vi "Save Data To File.vi"(7 "Data Type (0: Limit Test Data)":i32(ring) items=["Limit Test Data", "Math Expression Data", "Sense Data", "All Data"], 8 "error in (no error)":errorcluster, 9 "File Name":string, 10 "Channel (1: Channel 1)":i32(ring)=1 items=["Channel 1"=1], 11 "VISA resource name":refnum<visa-resource-name>) -> (0 "error out":errorcluster, 3 "VISA resource name out":refnum<visa-resource-name>)   [LabVIEW 2012, in "Keysight B2980 Series.lvlib"]
doc: "Saves the limit test data, math expression result data, sense data, or all of these data for the specified channel to the specified file in the current directory."
uses:
  Keysight B2980 Series.lvlib
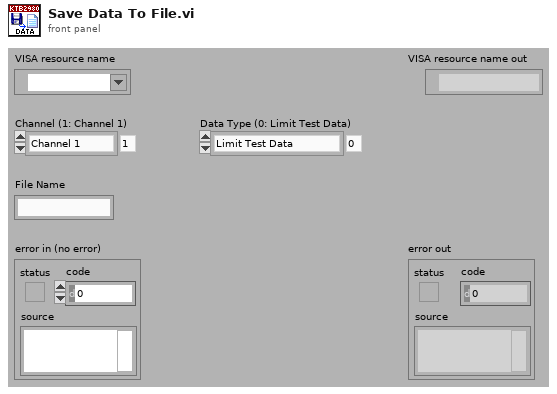
[diagram p1: front panel]
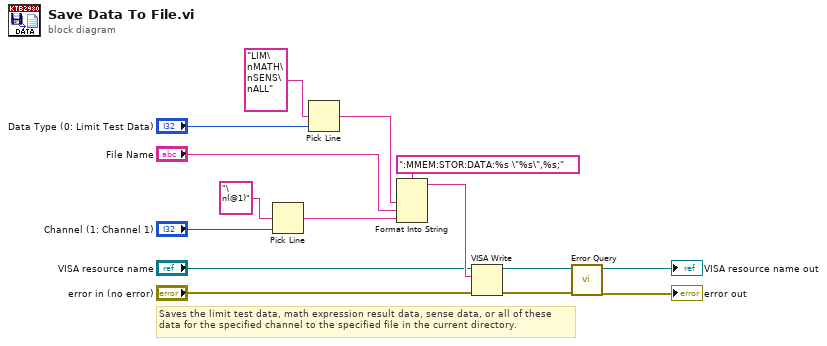
[diagram p0: block diagram]
diagram:
  # "Saves the limit test data, math expression result data, sense data, or all of these \ndata for the specified channel to the specified file in the current directory."
  n1 = Pick Line(multi-line string="\n(@1)", line index="Channel (1: Channel 1)") -> (output string=w1:string)  [unwired: 1 out]
  n2 = Pick Line(multi-line string="LIM\nMATH\nSENS\nALL", line index="Data Type (0: Limit Test Data)") -> (output string=w12:string)  [unwired: 1 out]
  n3 = Format Into String(format string=":MMEM:STOR:DATA:%s \"%s\",%s;", w12, "File Name", w1) -> (resulting string=w10:string)  [unwired: 2 in, 1 out]
  n4 = VISA Write(VISA resource name="VISA resource name", write buffer=w10, error in (no error)="error in (no error)") -> (VISA resource name out=w7:refnum<visa-resource-name>, error out=w6:errorcluster)  [unwired: 1 out]
  n5 = call "Error Query.vi"("error in (no error)"=w6, "VISA resource name"=w7) -> ("error out"=→"error out":errorcluster, "VISA resource name out"=→"VISA resource name out":refnum<visa-resource-name>)  [unwired: 8 out]
